vi "acquireAndDetectTest-OpenVINO.vi"() -> ()   [LabVIEW 2024]
uses:
  src/elements/black-squircle-dropdown.ctl
  src/elements/black-squircle-ring.ctl
  <vilib>/vision/Deep Learning.llb/IMAQ DL Model Output Data.ctl
  <vilib>/vision/Image Controls.llb/IMAQ Image.ctl
  <vilib>/userDefined/High Color/IMAQdx.ctl
  <vilib>/vision/Deep Learning.llb/IMAQ DL Model Label.ctl
  <vilib>/Utility/error.llb/DialogType.ctl
  <vilib>/vision/driver/IMAQdx.llb/IMAQdx Buffer Number Mode.ctl
  <vilib>/vision/driver/IMAQdx.llb/IMAQdx Acquisition Mode.ctl
  src/toolkit/rectangularDetectedObject.ctl
  <resource>/objmgr/imaqdx.rc
  <vilib>/vision/driver/NI_Vision_Acquisition_Software.lvlib
  src/toolkit/transformCv.lvclass
  <vilib>/vision/NI_Vision_Development_Module.lvlib
panel:
  out "error status":string
  out "fps":dbl format="%.1g FPS"
  in  "or ct":i32=5 caption="Orange Count"
  in  "sb ct":i32=5 caption="Starburst Count"
  in  "ro ct":i32=5 caption="Rollo Count"
  in  "update":bool
  in  "res":T1 caption="Resolution:" items=["160x120 YUY2 30.00fps", "320x180 YUY2 30.00fps", "320x240 YUY2 30.00fps", "424x240 YUY2 30.00fps", "640x360 MJPG 30.00fps", "640x360 YUY2 30.00fps", "640x480 MJPG 30.00fps", "640x480 YUY2 30.00fps", "848x480 MJPG 30.00fps", "960x540 MJPG 30.00fps", "1280x720 MJPG 30.00fps"]
  in  "pause":bool
  in  "play":bool
  in  "cam":T2 caption="Camera:"
  out "img":T3(plugin-control)
  out "Output Data Array":T4[](array[typedef]) {"Data" format="%#_2f"}
  out "proc time":dbl caption="Processing Time:" format="%.1p"
  out "pps":i32 caption="Parts per Second:"
  out "parts":i32 caption="Total Parts:"
  out "p/f":string="PASS / FAIL"
  out "or def":i32 caption="Rollos"
  out "sb def":i32 caption="Rollos"
  out "ro def":i32 caption="Rollos"
  out "or":i32 caption="Oranges"
  out "sb":i32 caption="Starbursts"
  out "ro":i32 caption="Rollos"
  out "or%":dbl caption="Rollos" format="%.1g%"
  out "sb%":dbl caption="Rollos" format="%.1g%"
  out "ro%":dbl caption="Rollos" format="%.1g%"
  # "Ct."
  # "Def."
  # "Conf."
  # "Transform-CV Acquire and Detect Demo v1.0.0"
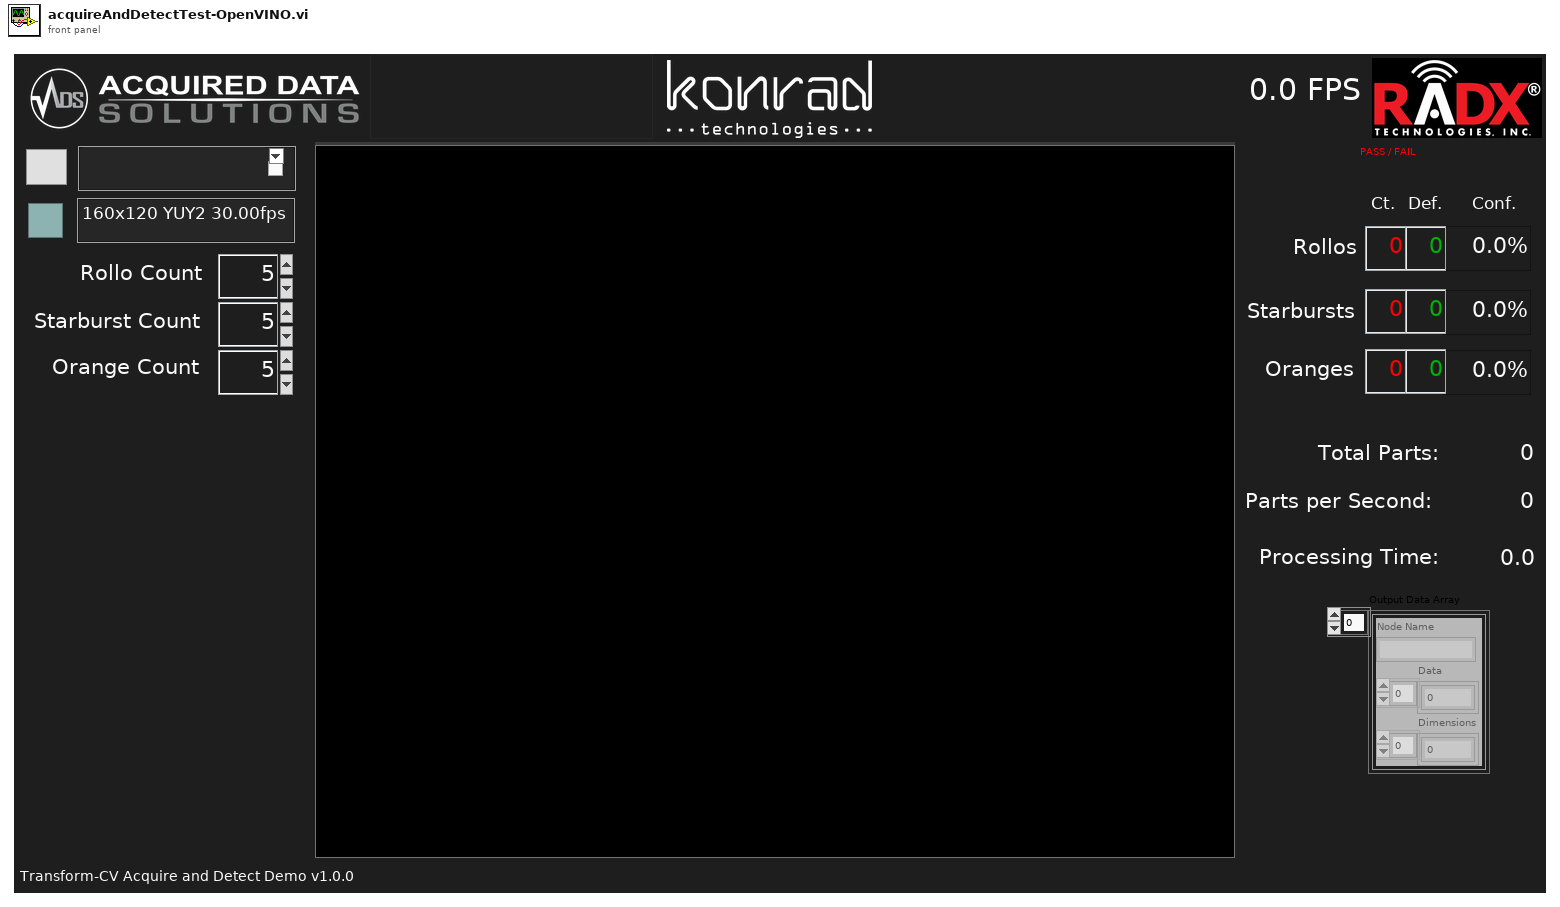
[diagram p1: front panel]
types:
  T1 = typedef "black-squircle-ring.ctl" = u16
  T2 = typedef "black-squircle-dropdown.ctl" = string
  T3 = typedef "IMAQ Image.ctl" = refnum<image>
  T4 = typedef "IMAQ DL Model Output Data.ctl" = cluster{"Node Name":string, "Data":sgl[], "Dimensions":u64[]}
  T5 = typedef "IMAQ DL Model Label.ctl" = cluster{"ID":u32, "Label":string}
  T6 = typedef "IMAQdx.ctl" = refnum<k21>
  T7 = typedef "IMAQ DL Model Refnum.ctl" = refnum<k20>
  T8 = typedef "NI_Vision_Acquisition_Software.lvlib/IMAQdx Buffer Number Mode.ctl" = enum32{"Next", "Last", "Buffer Number", "Every", "Last New"}
  T9 = typedef "NI_Vision_Acquisition_Software.lvlib/IMAQdx Acquisition Mode.ctl" = enum32{"One Shot", "Continuous"}
  T10 = typedef "DialogType.ctl" = u16
  T11 = typedef "transformCv.lvclass/rectangularDetectedObject.ctl" = cluster{"x1":sgl, "y1":sgl, "x2":sgl, "y2":sgl, "conf":sgl, "cls":i32}
  T12 = cluster{"good ct":i32, "bad ct":i32, "avg conf":dbl}[]
  T13 = cluster{"good ct":i32, "bad ct":i32, "avg conf":dbl}
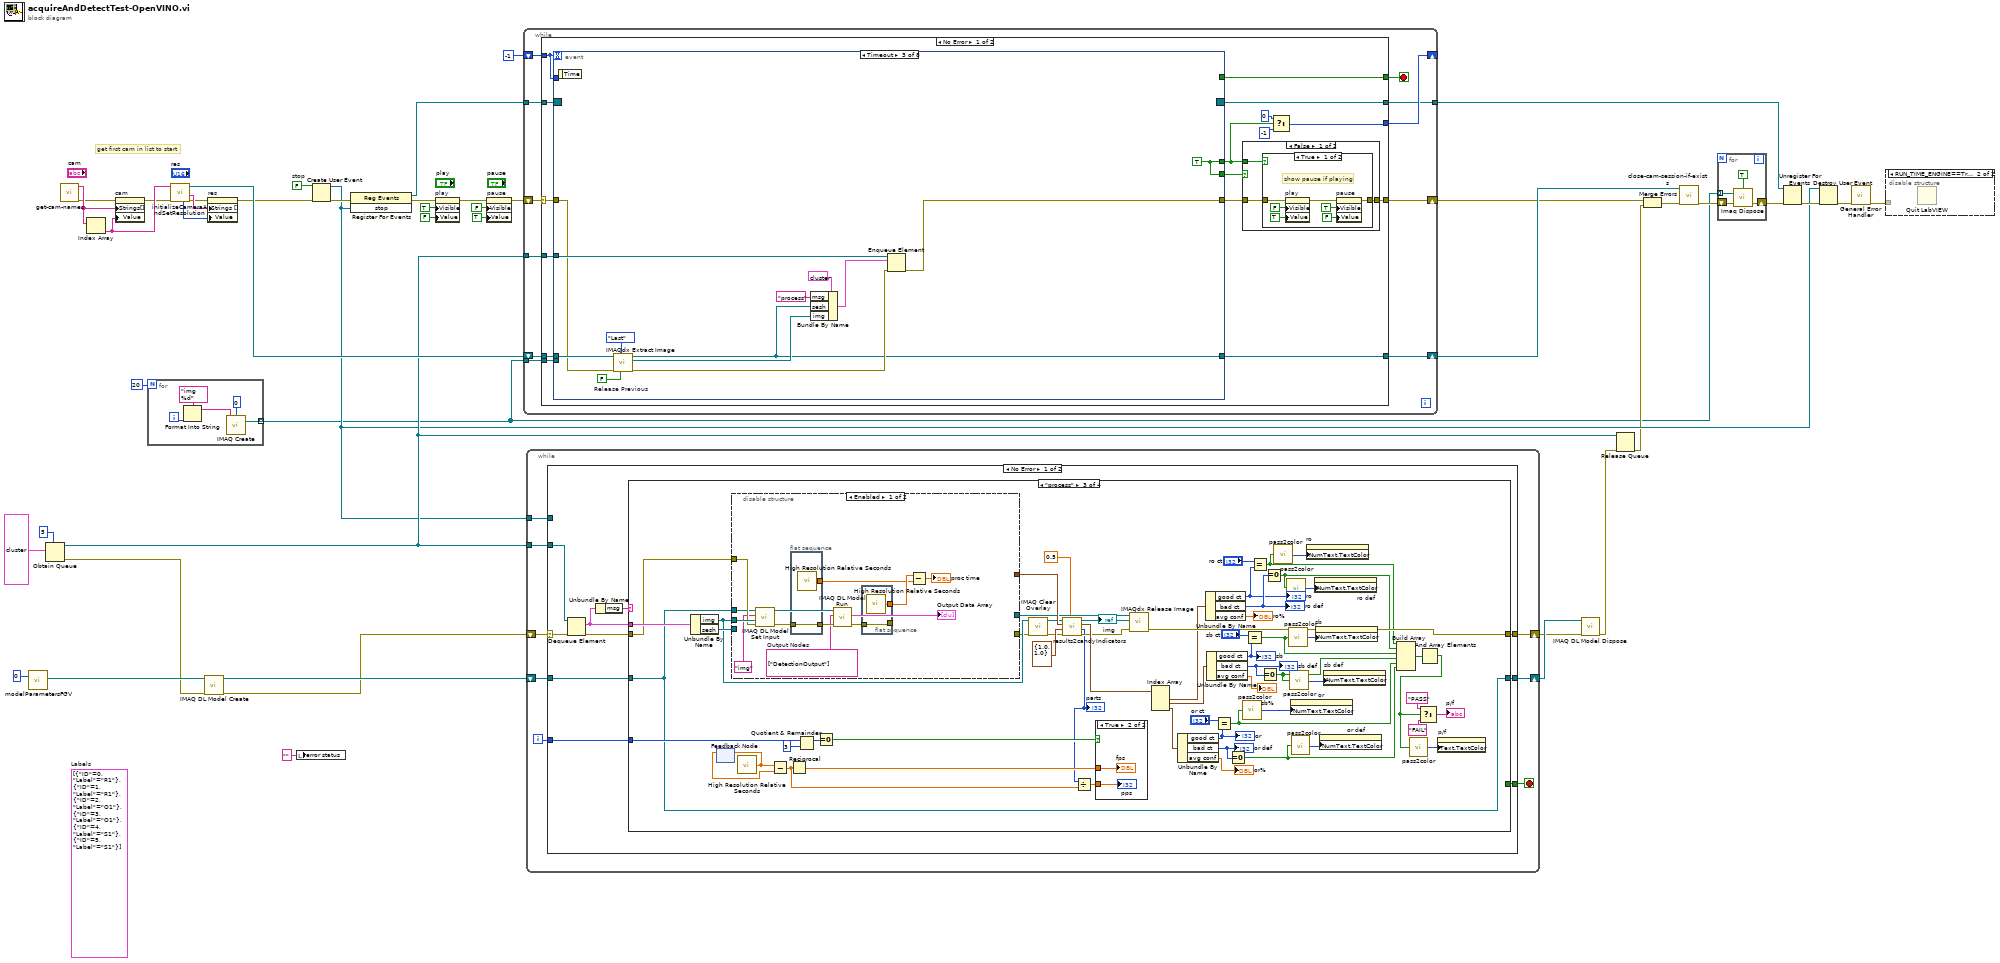
[diagram p0: block diagram]
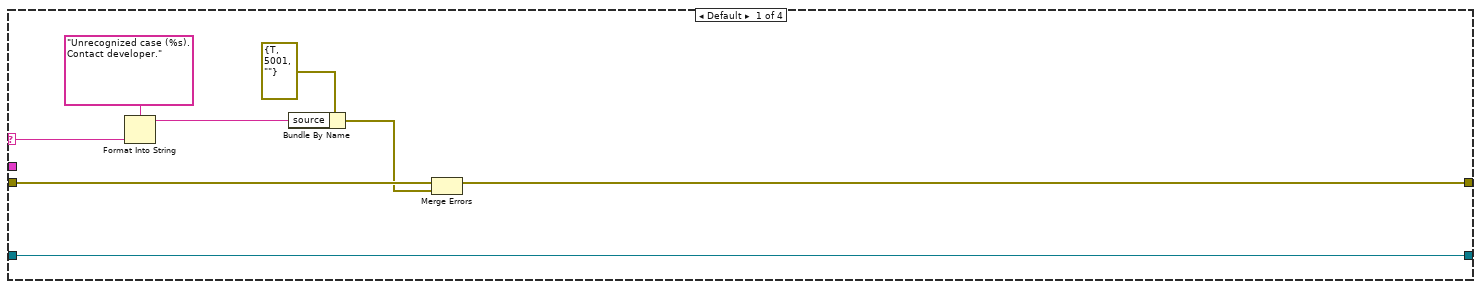
[diagram p2: hidden frame]
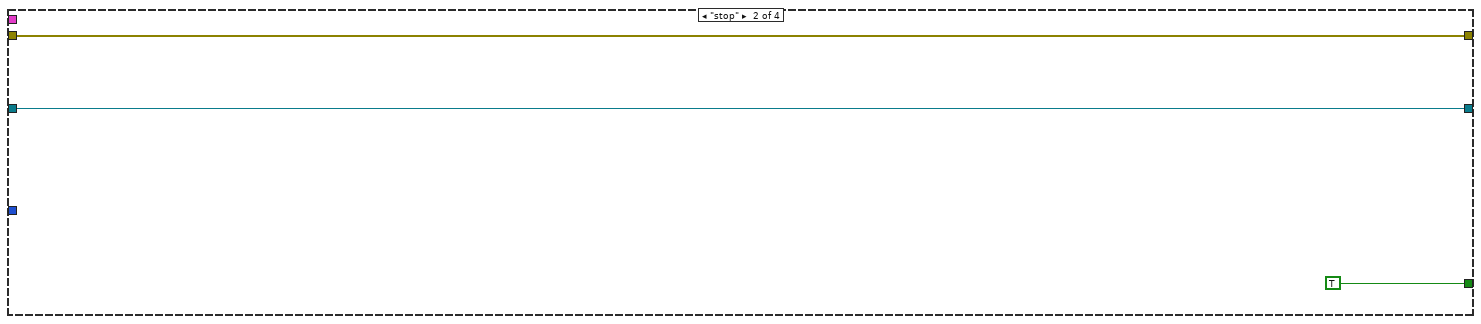
[diagram p3: hidden frame]
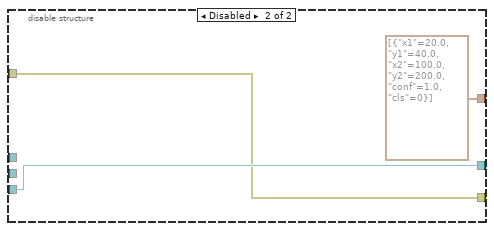
[diagram p4: hidden frame]
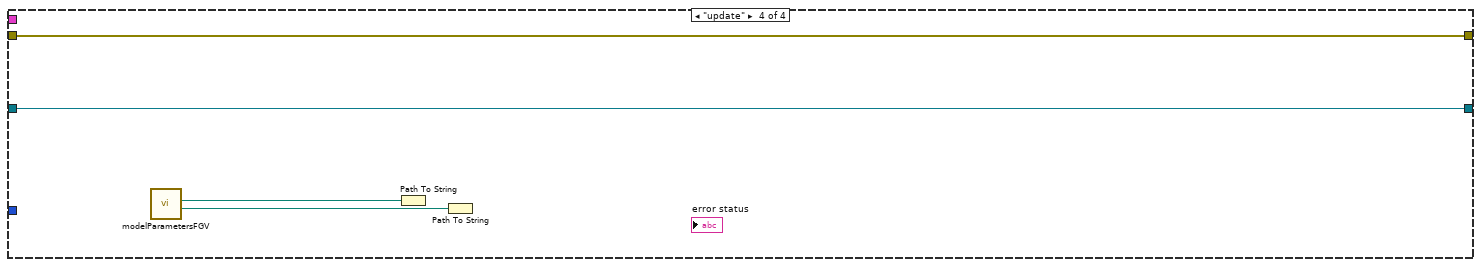
[diagram p6: hidden frame]
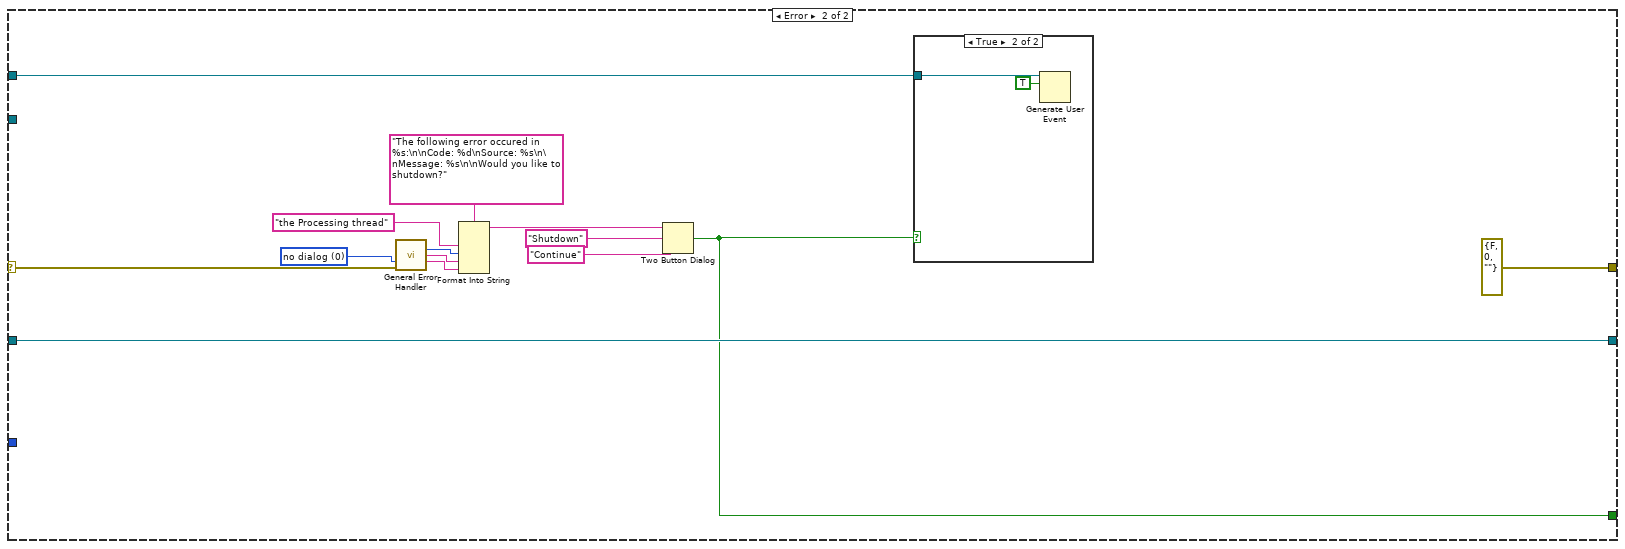
[diagram p7: hidden frame]
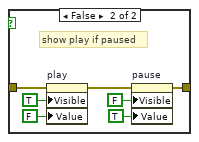
[diagram p10: hidden frame]
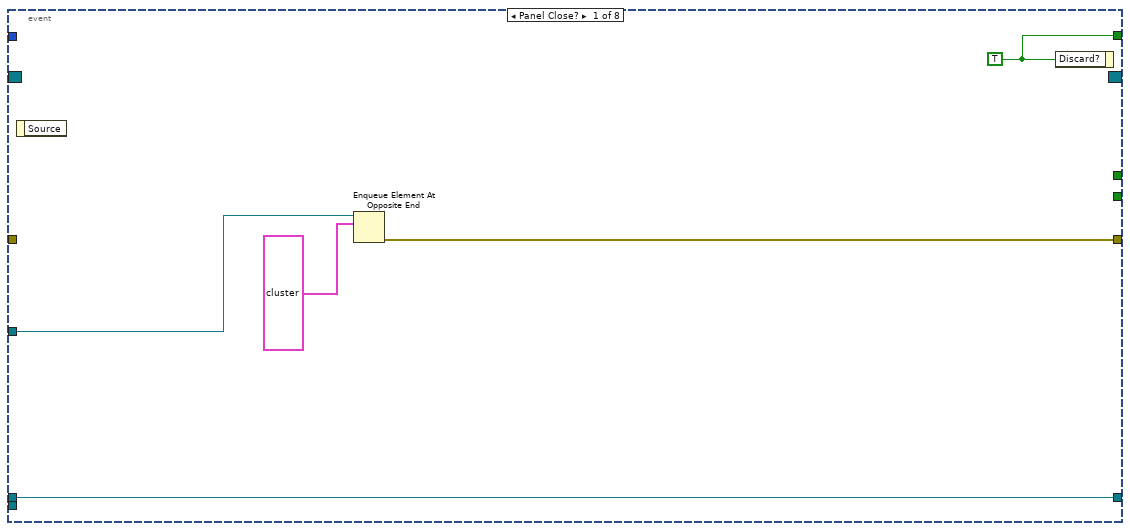
[diagram p12: hidden frame]
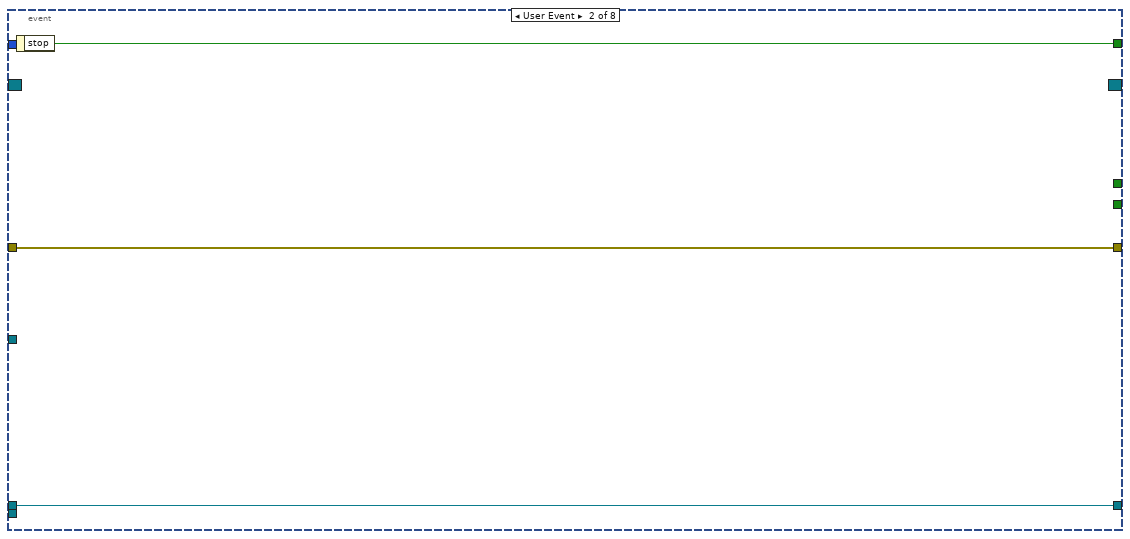
[diagram p13: hidden frame]
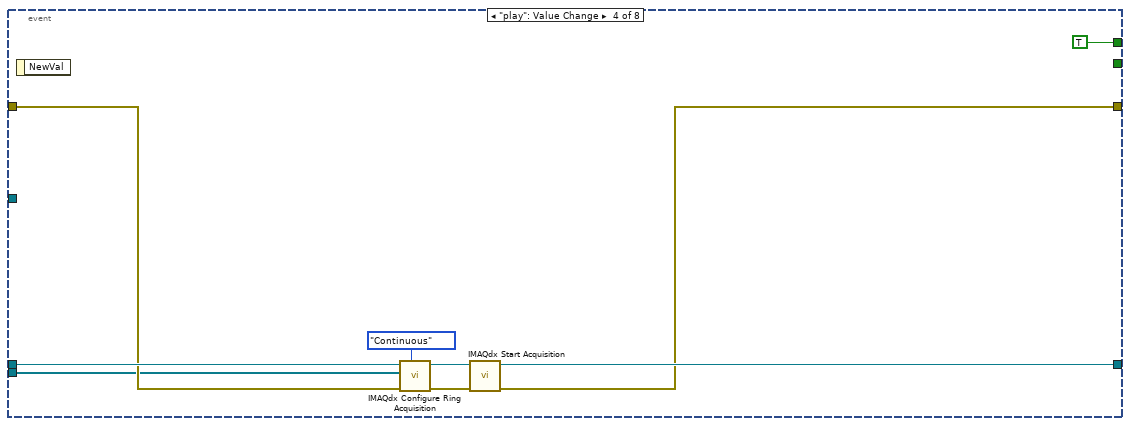
[diagram p14: hidden frame]
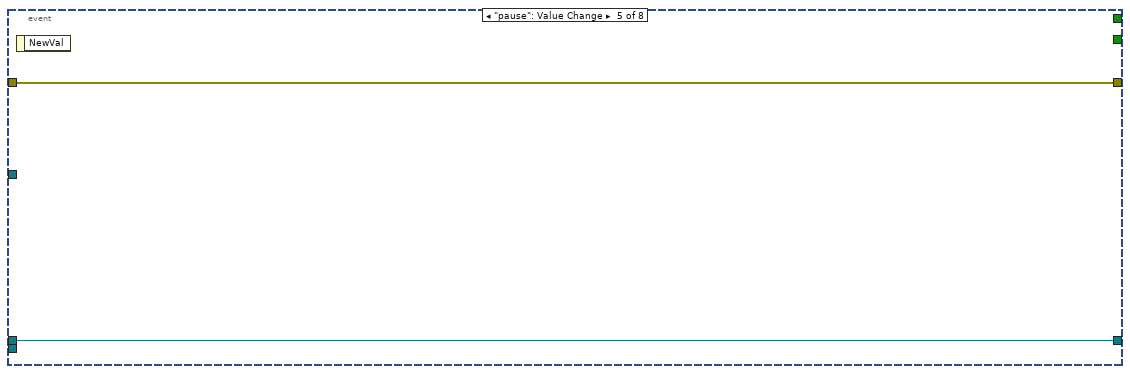
[diagram p15: hidden frame]
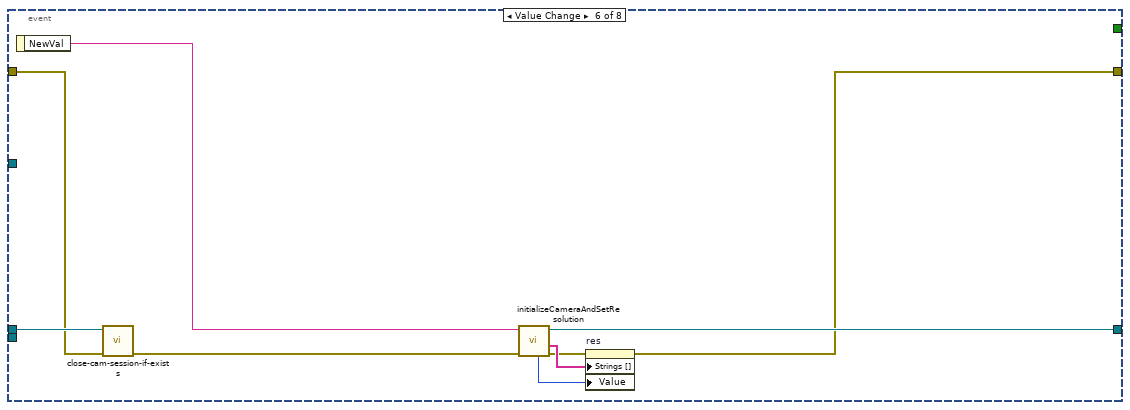
[diagram p16: hidden frame]
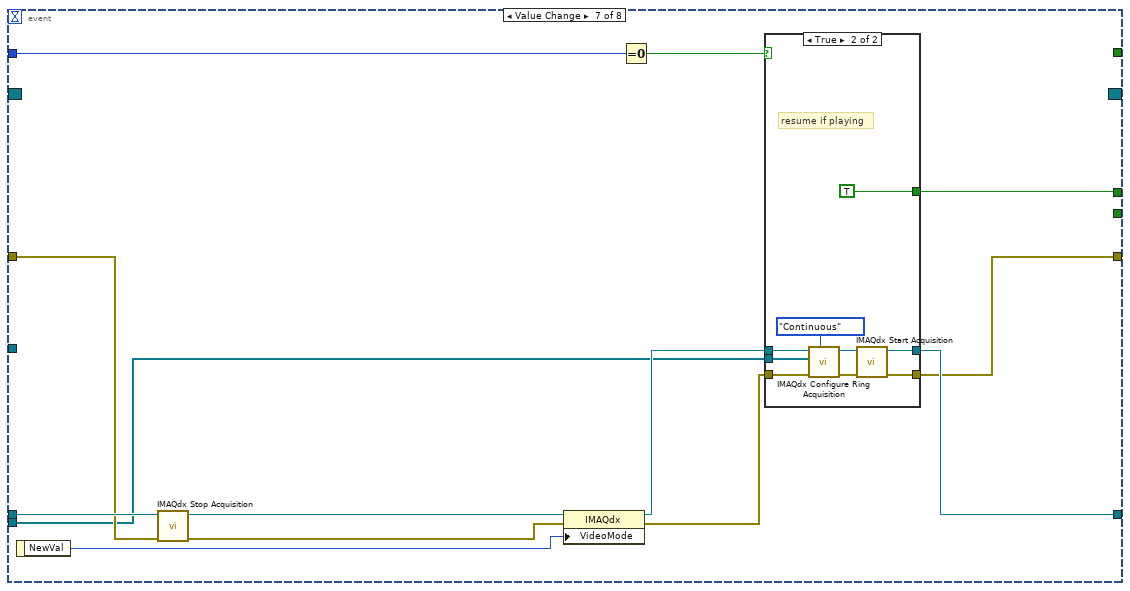
[diagram p17: hidden frame]
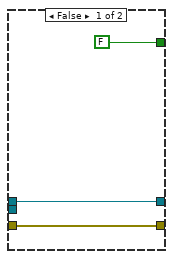
[diagram p18: hidden frame]
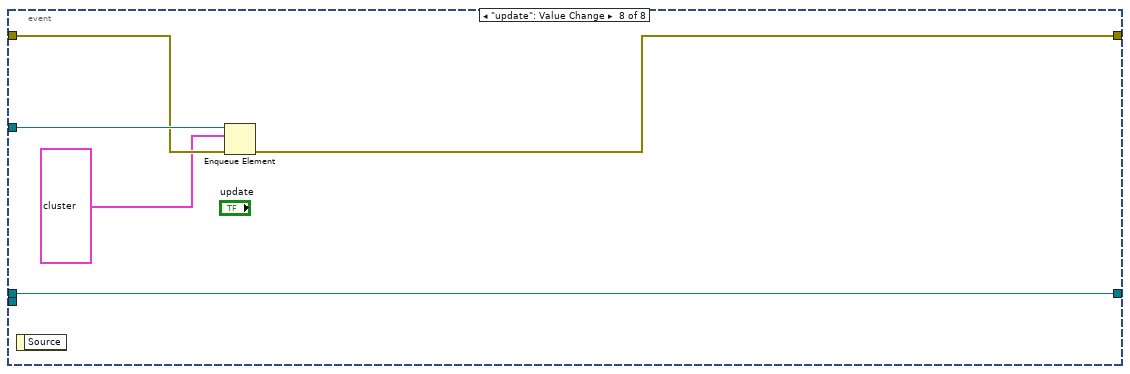
[diagram p19: hidden frame]
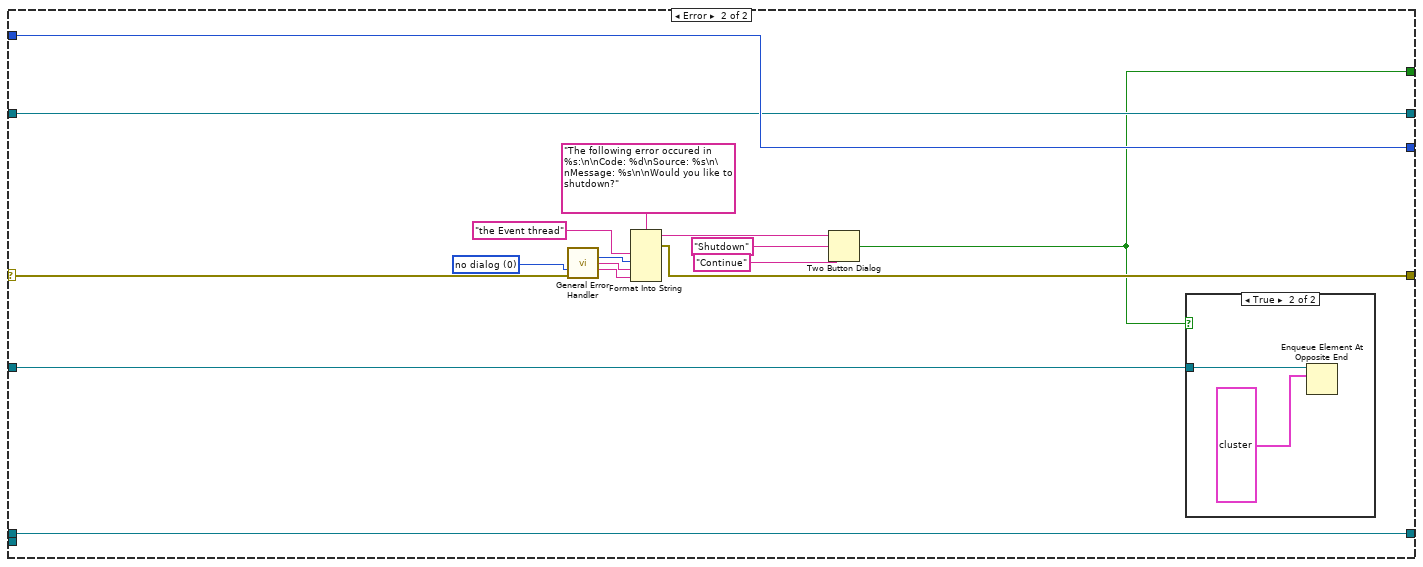
[diagram p20: hidden frame]
diagram:
  (unwired) T5[] [{"ID"=0, "Label"="R1"}, {"ID"=1, "Label"="R1"}, {"ID"=2, "Label"="O1"}, {"ID"=3, "Label"="O1"}, {"ID"=4, "Label"="S1"}, {"ID"=5, "Label"="S1"}]  # Labels
  w25 = FALSE  # stop
  # "get first cam in list to start"
  n1 = call "modelParametersFGV.vi"("timeout (-1)"=0) -> ("model out"=w8:path)  [unwired: 3 in, 3 out]
  n2 = Obtain Queue(max queue size (-1, unlimited)=5, element data type=cluster{"msg":string, "img":T3, "sesh":T6} {"msg"="", "img"=refnum, "sesh"=""}) -> (queue out=w28:refnum<queue>, error out=w7:errorcluster)  [unwired: 3 in, 1 out]
  n3 = call "get-cam-names.vi"() -> ("error out"=w31:errorcluster, "cam names"=w38:string[])  [unwired: 10 in]
  n4 = Index Array(array=w38) -> (element=w37:string)  [unwired: 1 in]
  n5 = property on="cam" class="CmbBox (strict)"(error in=w31, "Strings[]"=w38, "Value"=w37) -> (error out=w36:errorcluster)  [unwired: 1 in, 1 out]
  n6 = for {
    N: 20 -> [_]
    tunnel: [w50] -> w11 mode=indexing
    i -> [w49]
    n7 = Format Into String(format string="img %d" ("Image Name"), w49) -> (resulting string=w48:string)  [unwired: 2 in, 1 out]
    n8 = call "IMAQ Create"("Border Size"=0, "Image Name"=w48) -> ("New Image"=w50:T3)  [unwired: 2 in, 2 out]
  }
  n9 = call "initializeCameraAndSetResolution.vi"("error in"=w36, "seesion in"=w37) -> ("error out"=w33:errorcluster, "mode names"=w35:string[], "session out"=w32:T6, "current mode"=w34:u32)  [unwired: 5 in, 1 out]
  n10 = call-poly "IMAQ DL Model Create"("error in (no error)"=w7, "File Path"=w8) -> ("error out"=w2:errorcluster, "Model Refnum"=w6:T7)  [unwired: 8 in]
  n11 = property on="res" class="Ring (strict)"(error in=w33, "Strings []"=w35, "Value"=w34) -> (error out=w24:errorcluster)  [unwired: 1 in, 1 out]
  n12 = local write "error status"("" ("error status")) -> ()
  n13 = Create User Event(user event datatype=w25, error in=w24) -> (user event=w17:refnum<user-event>, error out=w26:errorcluster)
  n14 = register-events(error in=w26, w17) -> (reference out=w21:refnum<event-registration>, error out=w27:errorcluster)  [unwired: 1 in]
  n15 = property on="play" class="Bool (strict)"(error in=w27, "Visible"=TRUE, "Value"=FALSE ("play")) -> (error out=w43:errorcluster)  [unwired: 1 in, 1 out]
  n16 = property on="pause" class="Bool (strict)"(error in=w43, "Visible"=FALSE, "Value"=TRUE ("Visible")) -> (error out=w44:errorcluster)  [unwired: 1 in, 1 out]
  n17 = while {
    shift-right: [w61] -> w14
    shift-left: w44 -> [w60]
    shift-right: [w57] -> _
    shift-left: -1 -> [w58]
    shift-right: [w55] -> w22
    shift-left: w32 -> [w56]
    tunnel: w11 -> [w54]
    tunnel: w28 -> [w53]
    tunnel: w21 -> [w52]
    tunnel: [w51] -> w19
    stop <- w59 stop-if-true
    n18 = case shown="No Error" w60 {
      selector: w60 -> [w77 w174]
      tunnel: [w71 w173] -> w61
      tunnel: [w76 w167] -> w59
      tunnel: w58 -> [w65 w171]
      tunnel: [w73 w171] -> w57
      tunnel: w56 -> [w68 w170]
      tunnel: [w67 w170] -> w55
      tunnel: w54 -> [w66 _]
      tunnel: w53 -> [w64 w168]
      tunnel: w52 -> [w63 w169]
      tunnel: [w62 w169] -> w51
      frame No Error {
        n19 = event shown="[2] Timeout" {
          selector: w63 -> [_ _ _ _ _ _ _ _]
          dyn-events: [_ _ _ _ _ _ _ _] -> w62
          timeout: w65 -> [_ _ _ _ _ _ _ _]
          tunnel: w77 -> [_ w102 w109 w120 w127 w130 w146 w164]
          tunnel: [w100 w103 _ _ _ _ _ _] -> w76
          tunnel: [w99 w102 w112 w118 w127 w128 w139 w163] -> w72
          tunnel: [_ _ w116 TRUE ("s") _ _ w138 _] -> w70
          tunnel: [_ _ w116 _ _ _ _ _] -> w69
          tunnel: w68 -> [w97 w101 w110 w121 w126 w131 w148 w166]
          tunnel: [w97 w101 w104 w119 w126 w135 w140 w166] -> w67
          tunnel: w66 -> [_ _ _ w117 _ _ w137 _]
          tunnel: w65 -> [_ _ _ _ _ _ w144 _]
          tunnel: w64 -> [w98 _ w115 _ _ _ _ w165]
          event Panel Close? {
            w100 = TRUE ("Discard?")
            n20 = event-data() -> ()  [unwired: 1 in, 1 out]
            n21 = Enqueue Element At Opposite End(queue=w98, element=cluster{"msg":string, "img":T3, "sesh":T6} {"msg"="stop", "img"=refnum, "sesh"=""}) -> (error out=w99:errorcluster)  [unwired: 2 in, 2 out]
            n22 = event-data("Discard?"=w100) -> ()  [unwired: 1 in, 1 out]
          }
          event User Event {
            n23 = event-data() -> ("stop"=w103:bool)  [unwired: 1 in]
          }
          event Timeout {
            w108 = FALSE  # Release Previous
            w116 = TRUE ("s")
            n24 = event-data() -> ()  [unwired: 1 in, 1 out]
            n25 = call <vilib>:"IMAQdx Extract Image.vi"("Release Previous (true)"=w108, "Buffer Number Mode (Next)"=IMAQdx_Buffer_Number_Mode."Last" ("Buffer Number Mode"), "error in"=w109, "Session In"=w110) -> ("error out"=w105:errorcluster, "Image Out"=w106:T3, "Session Out"=w104:T6)  [unwired: 4 in, 1 out]
            n26 = Bundle By Name(cluster=cluster{"msg":string, "img":T3, "sesh":T6} {"msg"="", "img"=refnum, "sesh"=""}, "msg"="process", "sesh"=w104, "img"=w106) -> (w113:cluster{"msg":string, "img":T3, "sesh":T6})
            n27 = Enqueue Element(queue=w115, element=w113, error in (no error)=w105) -> (error out=w112:errorcluster)  [unwired: 1 in, 2 out]
          }
          event "play": Value Change {
            n28 = event-data() -> ()  [unwired: 1 in, 1 out]
            n29 = call <vilib>:"IMAQdx Configure Ring Acquisition.vi"("Mode"=IMAQdx_Acquisition_Mode."Continuous" ("Continuous?"), "error in"=w120, "Images"=w117, "Session In"=w121) -> ("error out"=w123:errorcluster, "Session Out"=w124:T6)  [unwired: 5 in, 1 out]
            n30 = call <vilib>:"IMAQdx Start Acquisition.vi"("error in"=w123, "Session In"=w124) -> ("error out"=w118:errorcluster, "Session Out"=w119:T6)  [unwired: 8 out]
          }
          event "pause": Value Change {
            n31 = event-data() -> ()  [unwired: 1 in, 1 out]
          }
          event Value Change {
            n32 = event-data() -> ("NewVal"=w136:T2)  [unwired: 1 in]
            n33 = call "close-cam-session-if-exists.vi"("error in (no error)"=w130, "cam in"=w131) -> ("error out"=w129:errorcluster)  [unwired: 9 in]
            n34 = call "initializeCameraAndSetResolution.vi"("error in"=w129, "seesion in"=w136) -> ("error out"=w133:errorcluster, "mode names"=w134:string[], "session out"=w135:T6, "current mode"=w132:u32)  [unwired: 5 in, 1 out]
            n35 = property on="res" class="Ring (strict)"(error in=w133, "Strings []"=w134, "Value"=w132) -> (error out=w128:errorcluster)  [unwired: 1 in, 1 out]
          }
          event Value Change {
            n36 = event-data() -> ("NewVal"=w149:T1)  [unwired: 1 in]
            n37 = call <vilib>:"IMAQdx Stop Acquisition.vi"("error in"=w146, "Session In"=w148) -> ("error out"=w145:errorcluster, "Session Out"=w147:T6)  [unwired: 8 in]
            n38 = property class="IMAQdx"(reference=w147, error in=w145, "VideoMode"=w149) -> (reference out=w142:T6, error out=w141:errorcluster)
            n39 = Equal To 0?(x=w144) -> (x = 0?=w143:bool)
            n40 = case shown="True" w143 {
              tunnel: w142 -> [w151 w157]
              tunnel: w141 -> [w150 w155]
              tunnel: [w151 w156] -> w140
              tunnel: [w150 w154] -> w139
              tunnel: [FALSE ("s") TRUE ("s")] -> w138
              tunnel: w137 -> [_ w153]
              frame False {
              }
              frame True {
                # "resume if playing"
                n41 = call <vilib>:"IMAQdx Configure Ring Acquisition.vi"("Mode"=IMAQdx_Acquisition_Mode."Continuous" ("Continuous?"), "error in"=w155, "Images"=w153, "Session In"=w157) -> ("error out"=w160:errorcluster, "Session Out"=w159:T6)  [unwired: 5 in, 1 out]
                n42 = call <vilib>:"IMAQdx Start Acquisition.vi"("error in"=w160, "Session In"=w159) -> ("error out"=w154:errorcluster, "Session Out"=w156:T6)  [unwired: 8 out]
              }
            }
          }
          event "update": Value Change {
            n43 = event-data() -> ()  [unwired: 1 in, 1 out]
            n44 = Enqueue Element(queue=w165, element=cluster{"msg":string, "img":T3, "sesh":T6} {"msg"="update", "img"=refnum, "sesh"=""}, error in (no error)=w164) -> (error out=w163:errorcluster)  [unwired: 1 in, 2 out]
          }
        }
        n45 = case shown="False" w69 {
          tunnel: w72 -> [w80 w95]
          tunnel: [w79 w95] -> w71
          tunnel: w70 -> [w78 _]
          frame False {
            n46 = case shown="True" w78 {
              tunnel: w80 -> [w82 w89]
              tunnel: [w81 w88] -> w79
              frame True {
                # "show pause if playing"
                n47 = property on="play" class="Bool (strict)"(error in=w82, "Visible"=FALSE, "Value"=TRUE ("play")) -> (error out=w84:errorcluster)  [unwired: 1 in, 1 out]
                n48 = property on="pause" class="Bool (strict)"(error in=w84, "Visible"=TRUE, "Value"=FALSE ("Visible")) -> (error out=w81:errorcluster)  [unwired: 1 in, 1 out]
              }
              frame False {
                # "show play if paused"
                n49 = property on="play" class="Bool (strict)"(error in=w89, "Visible"=TRUE, "Value"=FALSE ("play")) -> (error out=w91:errorcluster)  [unwired: 1 in, 1 out]
                n50 = property on="pause" class="Bool (strict)"(error in=w91, "Visible"=FALSE, "Value"=TRUE ("Visible")) -> (error out=w88:errorcluster)  [unwired: 1 in, 1 out]
              }
            }
          }
          frame True {
            # "don't waste time on update if running continuous acquisition"
          }
        }
        n51 = Select(t=0, s=w70, f=-1) -> (s? t:f=w73:i32)
      }
      frame Error {
        w182 = T10 0 items=["no dialog", "OK message", "continue or stop message", "OK message + warnings", "continue/stop + warnings"] ("type of dialog (OK msg:1)")
        n52 = call <vilib>:"General Error Handler.vi"("type of dialog (OK msg:1)"=w182, "error in (no error)"=w174) -> ("code out"=w175:i32, "source out"=w177:string, "message"=w178:string)  [unwired: 9 in, 2 out]
        n53 = Format Into String(format string="The following error occured in %s:\n\nCode: %d\nSource: %s\n\nMessage: %s\n\nWould you like to shutdown?", "the Event thread" ("input 1"), w175, w177, w178) -> (resulting string=w179:string, error out=w173:errorcluster)  [unwired: 2 in]
        n54 = Two Button Dialog(message=w179, 1:"Continue" ("F button name (\"Cancel\")"), 2:"Shutdown" ("T button name (\"OK\")")) -> (T button?=w167:bool)
        n55 = case shown="True" w167 {
          tunnel: w168 -> [_ w183]
          frame False {
          }
          frame True {
            n56 = Enqueue Element At Opposite End(queue=w183, element=cluster{"msg":string, "img":T3, "sesh":T6} {"msg"="stop", "img"=refnum, "sesh"=""}) -> ()  [unwired: 2 in, 3 out]
          }
        }
      }
    }
  }
  n57 = while {
    shift-right: [w188] -> w4
    shift-left: w2 -> [w192]
    shift-right: [w190] -> w5
    shift-left: w6 -> [w191]
    tunnel: w28 -> [w189]
    tunnel: w17 -> [w187]
    i -> [w185]
    stop <- w186 stop-if-true
    n58 = case shown="No Error" w192 {
      selector: w192 -> [w202 w304]
      tunnel: w191 -> [w197 w303]
      tunnel: [w195 w303] -> w190
      tunnel: w189 -> [w201 _]
      tunnel: [w199 errorcluster {"status"=FALSE, "code"=0, "source"=""} ("error out")] -> w188
      tunnel: w187 -> [_ w300]
      tunnel: [w194 w301] -> w186
      tunnel: w185 -> [w193 _]
      frame No Error {
        n59 = Dequeue Element(queue=w201, error in (no error)=w202) -> (element=w196:cluster{"msg":string, "img":T3, "sesh":T6}, error out=w198:errorcluster)  [unwired: 1 in, 2 out]
        n60 = Unbundle By Name(w196) -> ("msg"=w200:string)
        n61 = case shown="\"process\"" w200 {
          selector: w200 -> [w210 _ _ _]
          tunnel: [w203 w212 w266 w296] -> w199
          tunnel: w198 -> [w205 w212 w216 w296]
          tunnel: w197 -> [w206 w213 w215 w297]
          tunnel: w196 -> [_ _ w270 _]
          tunnel: [w206 w213 w215 w297] -> w195
          tunnel: [_ TRUE _ _] -> w194
          tunnel: w193 -> [_ _ w265 _]
          frame Default {
            n62 = Format Into String(format string="Unrecognized case (%s). Contact developer.", w210) -> (resulting string=w207:string)  [unwired: 2 in, 1 out]
            n63 = Bundle By Name(cluster=errorcluster {"status"=TRUE, "code"=5001, "source"=""} ("error constant"), "source"=w207) -> (w204:errorcluster)
            n64 = Merge Errors(w205, w204) -> (w203:errorcluster)
          }
          frame "stop" {
          }
          frame "process" {
            n65 = Unbundle By Name(w270) -> ("img"=w258:T3, "sesh"=w269:T6)
            n66 = feedback #1() -> (w261:dbl)  [unwired: 1 in]
            n67 = disable-structure shown="Enabled" {
              disable-tunnel: [_ T11[] [{"x1"=20.0, "y1"=40.0, "x2"=100.0, "y2"=200.0, "conf"=1.0, "cls"=0}] ("results")] -> w272
              disable-tunnel: w269 -> [_ w293]
              disable-tunnel: [_ w293] -> w268
              disable-tunnel: w258 -> [w283 _]
              disable-tunnel: [_ w292] -> w256
              disable-tunnel: w216 -> [w282 w292]
              disable-tunnel: w215 -> [w281 _]
              frame Enabled {
                w275 = string[] ["DetectionOutput"]  # Output Nodes
                n68 = call-poly "IMAQ DL Model Set Input"("error in (no error)"=w282, "Image"=w283, "Input Node Name"="img", "Model Refnum In"=w281) -> ("error out"=w278:errorcluster, "Model Refnum Out"=w277:T7)  [unwired: 5 in, 1 out]
                n69 = flat-sequence {
                  tunnel: w278 -> [w290]
                  tunnel: [w290] -> w279
                  tunnel: [w289] -> w285
                  frame #0 {
                    n70 = call <vilib>:"High Resolution Relative Seconds.vi"() -> ("relative seconds"=w289:dbl)
                  }
                }
                n71 = call "IMAQ DL Model Run"("error in (no error)"=w279, "Output Node Names"=w275, "Model Refnum In"=w277) -> ("error out"=w276:errorcluster, "Output Data Array"=→"Output Data Array":T4[])  [unwired: 6 in, 1 out]
                n72 = flat-sequence {
                  tunnel: [w288] -> w286
                  tunnel: w276 -> [w287]
                  tunnel: [w287] -> _
                  frame #0 {
                    n73 = call <vilib>:"High Resolution Relative Seconds.vi"() -> ("relative seconds"=w288:dbl)
                  }
                }
                n74 = Subtract(x=w286, y=w285) -> (x-y=→"proc time":dbl)
              }
              frame Disabled {
              }
            }
            n75 = call <vilib>:"High Resolution Relative Seconds.vi"() -> ("relative seconds"=w262:dbl)
            n76 = feedback-in #1(w262) -> ()
            n77 = Subtract(x=w262, y=w261) -> (x-y=w218:dbl)
            n78 = Reciprocal(x=w218) -> (1/x=w254:dbl)
            n79 = Quotient & Remainder(x=w265, y=3) -> (x-y*floor(x/y)=w263:i32)  [unwired: 1 out]
            n80 = Equal To 0?(x=w263) -> (x = 0?=w220:bool)
            n81 = call "IMAQ Clear Overlay"("error in (no error)"=w256, "Image"=w258) -> ("error out"=w255:errorcluster, "Image Out"=w257:T3)  [unwired: 8 in]
            n82 = call "results2candyIndicators.vi"("conf"=sgl 0.5, "error in (no error)"=w255, "scale"=cluster{"X":dbl, "Y":dbl} {"X"=1.0, "Y"=1.0}, "results"=w272, "img in"=w257) -> ("error out"=w259:errorcluster, "tot parts"=w219:i32, "ui array"=w273:T12, "img out"=w260:T3)  [unwired: 3 in]
            "img" <- w260
            "parts" <- w219
            n83 = Divide(x=w219, y=w218) -> (x/y=w217:dbl)
            n84 = case shown="True" w220 {
              tunnel: w254 -> [_ w295]
              tunnel: w217 -> [_ w294]
              frame False {
              }
              frame True {
                "fps" <- w295
                "pps" <- w294
              }
            }
            n85 = call <vilib>:"IMAQdx Release Image.vi"("error in"=w259, "Image"=w260, "Session In"=w268) -> ("error out"=w267:errorcluster)  [unwired: 7 in, 1 out]
            n86 = Index Array(array=w273) -> (element #1=w223:T13, element #2=w232:T13, element #3=w241:T13)  [unwired: 3 in]
            n87 = Unbundle By Name(w241) -> ("good ct"=w245:i32, "bad ct"=w247:i32, "avg conf"=→"or%":dbl)
            "or def" <- w247
            "or" <- w245
            n88 = Unbundle By Name(w223) -> ("good ct"=w224:i32, "bad ct"=w227:i32, "avg conf"=→"ro%":dbl)
            "ro" <- w224
            "ro def" <- w227
            n89 = Unbundle By Name(w232) -> ("good ct"=w237:i32, "bad ct"=w236:i32, "avg conf"=→"sb%":dbl)
            "sb def" <- w236
            "sb" <- w237
            n90 = Equal?(x="or ct", y=w245) -> (x = y?=w243:bool)
            n91 = Equal To 0?(x=w247) -> (x = 0?=w248:bool)
            n92 = call "pass2color.vi"("pass?"=w243) -> ("color"=w244:u32)
            n93 = Equal?(x="sb ct", y=w237) -> (x = y?=w235:bool)
            n94 = Equal?(x="ro ct", y=w224) -> (x = y?=w230:bool)
            n95 = Equal To 0?(x=w236) -> (x = 0?=w239:bool)
            n96 = Equal To 0?(x=w227) -> (x = 0?=w231:bool)
            n97 = call "pass2color.vi"("pass?"=w230) -> ("color"=w228:u32)
            n98 = call "pass2color.vi"("pass?"=w231) -> ("color"=w229:u32)
            n99 = call "pass2color.vi"("pass?"=w235) -> ("color"=w234:u32)
            n100 = call "pass2color.vi"("pass?"=w239) -> ("color"=w240:u32)
            n101 = property on="or" class="DigNum (strict)"("NumText.TextColor"=w244) -> ()  [unwired: 2 in, 2 out]
            n102 = call "pass2color.vi"("pass?"=w248) -> ("color"=w249:u32)
            n103 = property on="ro" class="DigNum (strict)"("NumText.TextColor"=w228) -> ()  [unwired: 2 in, 2 out]
            n104 = property on="ro def" class="DigNum (strict)"("NumText.TextColor"=w229) -> ()  [unwired: 2 in, 2 out]
            n105 = property on="sb" class="DigNum (strict)"(error in=w267, "NumText.TextColor"=w234) -> (error out=w266:errorcluster)  [unwired: 1 in, 1 out]
            n106 = property on="or def" class="DigNum (strict)"("NumText.TextColor"=w249) -> ()  [unwired: 2 in, 2 out]
            n107 = property on="sb def" class="DigNum (strict)"("NumText.TextColor"=w240) -> ()  [unwired: 2 in, 2 out]
            n108 = Build Array(w230, w231, w235, w239, w243, w248) -> (w250:bool[])
            n109 = And Array Elements(Boolean array=w250) -> (logical AND=w252:bool)
            n110 = call "pass2color.vi"("pass?"=w252) -> ("color"=w253:u32)
            n111 = Select(t="PASS" ("p/f"), s=w252, f="FAIL" ("p/f")) -> (s? t:f=→"p/f":string)
            n112 = property on="p/f" class="Str"("Text.TextColor"=w253) -> ()  [unwired: 2 in, 2 out]
          }
          frame "update" {
            n113 = call "modelParametersFGV.vi"() -> ("model out"=w298:path, "classes out"=w299:path)  [unwired: 4 in, 2 out]
            n114 = Path To String(path=w298) -> ()  [unwired: 1 out]
            n115 = Path To String(path=w299) -> ()  [unwired: 1 out]
          }
        }
      }
      frame Error {
        w305 = T10 0 items=["no dialog", "OK message", "continue or stop message", "OK message + warnings", "continue/stop + warnings"] ("type of dialog (OK msg:1)")
        n116 = call <vilib>:"General Error Handler.vi"("type of dialog (OK msg:1)"=w305, "error in (no error)"=w304) -> ("code out"=w312:i32, "source out"=w310:string, "message"=w309:string)  [unwired: 9 in, 2 out]
        n117 = Format Into String(format string="The following error occured in %s:\n\nCode: %d\nSource: %s\n\nMessage: %s\n\nWould you like to shutdown?", "the Processing thread" ("input 1"), w312, w310, w309) -> (resulting string=w308:string)  [unwired: 2 in, 1 out]
        n118 = Two Button Dialog(message=w308, 1:"Continue" ("F button name (\"Cancel\")"), 2:"Shutdown" ("T button name (\"OK\")")) -> (T button?=w301:bool)
        n119 = case shown="True" w301 {
          tunnel: w300 -> [_ w315]
          frame False {
          }
          frame True {
            n120 = Generate User Event(user event=w315, event data cluster=TRUE ("event data")) -> ()  [unwired: 2 in, 2 out]
          }
        }
      }
    }
  }
  n121 = call "IMAQ DL Model Dispose"("error in (no error)"=w4, "Model Refnum"=w5) -> ("error out"=w3:errorcluster)  [unwired: 9 in]
  n122 = Release Queue(queue=w28, error in (no error)=w3) -> (error out=w16:errorcluster)  [unwired: 1 in, 2 out]
  n123 = Merge Errors(w14, w16) -> (w13:errorcluster)
  n124 = call "close-cam-session-if-exists.vi"("error in (no error)"=w13, "cam in"=w22) -> ("error out"=w23:errorcluster)  [unwired: 9 in]
  n125 = for {
    tunnel: w11 -> [w316] mode=indexing
    shift-right: [w317] -> w20
    shift-left: w23 -> [w319]
    n126 = call "Imaq Dispose"("All Images? (No)"=TRUE, "Image"=w316, "error in (no error)"=w319) -> ("error out"=w317:errorcluster)  [unwired: 3 in]
  }
  n127 = Unregister For Events(event registration refnum=w19, error in=w20) -> (error out=w18:errorcluster)
  n128 = Destroy User Event(user event=w17, error in=w18) -> (error out=w12:errorcluster)
  n129 = call <vilib>:"General Error Handler.vi"("error in (no error)"=w12) -> ("error out"=w15:errorcluster)  [unwired: 10 in, 4 out]
  n130 = disable-structure shown="RUN_TIME_ENGINE==True" {
    disable-tunnel: w15 -> [_ _]
    frame condition #0 (active) {
    }
    frame condition #1 {
      n131 = Quit LabVIEW() -> ()  [unwired: 1 in]
    }
  }
